vi "Exemple 2.vi"() -> ()   [LabVIEW 2019, in "Minicircuit RF Switch Box.lvlib"]
uses:
  <instrlib>/Minicircuit RF Switch Box/Minicircuit RF Switch Box.lvlib
panel:
  in  "serial number":string
  out "Switch state":bool
  out "USB connection active?":bool
  in  "switch name":string
  in  "Switch state":bool
  out "error out":errorcluster
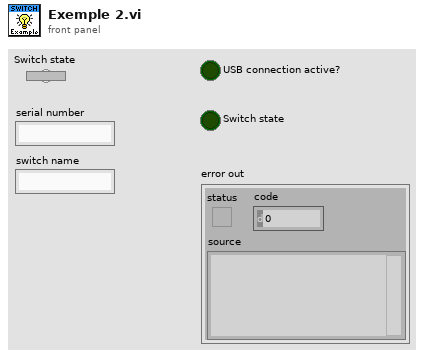
[diagram p1: front panel]
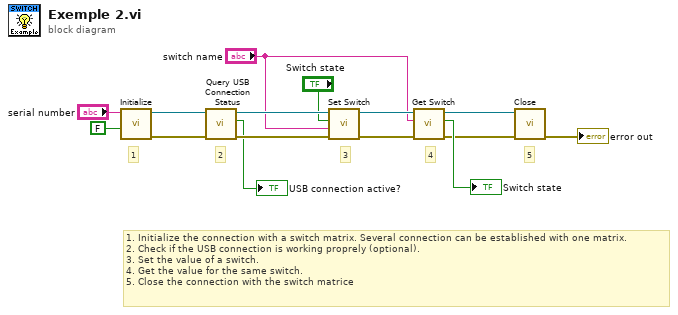
[diagram p0: block diagram]
diagram:
  # "3"
  # "1. Initialize the connection with a switch matrix. Several connection can be established with one matrix.\n2. Check if the USB connection is working proprely (optional).\n3. Set the value of a switch.\n4. Get the value for the same switch.\n5. Close the connection with the switch matrice"
  # "5"
  # "4"
  # "2"
  # "1"
  n1 = call <instrlib>:"Initialize.vi"("Reset (True)"=FALSE, "serial number"="serial number") -> ("error out"=w11:errorcluster, "MC switch refnum out"=w14:refnum<k24>)  [unwired: 8 in]
  n2 = call <instrlib>:"Query USB Connection Status.vi"("error in (no error)"=w11, "MC switch refnum in"=w14) -> ("error out"=w12:errorcluster, "USB connection active?"=→"USB connection active?":bool, "MC switch refnum out"=w13:refnum<k24>)  [unwired: 7 in]
  n3 = call <instrlib>:"Set Switch.vi"("error in (no error)"=w12, "switch name"="switch name", "value"="Switch state", "MC switch refnum in"=w13) -> ("error out"=w8:errorcluster, "MC switch refnum out"=w9:refnum<k24>)  [unwired: 6 in]
  n4 = call <instrlib>:"Get Switch.vi"("error in (no error)"=w8, "switch name"="switch name", "MC switch refnum in"=w9) -> ("error out"=w3:errorcluster, "state"=→"Switch state":bool, "MC switch refnum out"=w5:refnum<k24>)  [unwired: 6 in]
  n5 = call <instrlib>:"Close.vi"("error in (no error)"=w3, "MC switch refnum in"=w5) -> ("error out"=→"error out":errorcluster)  [unwired: 9 in]
